vi "create.vi"(8 "error in":errorcluster, 9 "Key":string, 10 "Upload ID":string) -> (0 "error out":errorcluster, 3 "Nominal Client MultiPart Upload":refnum<class "Multipart Upload.lvclass">)   [LabVIEW 2020, in "Multipart Upload.lvclass"]
uses:
  Multipart Upload.lvclass
  Multipart Upload.lvclass/Multipart Upload.ctl
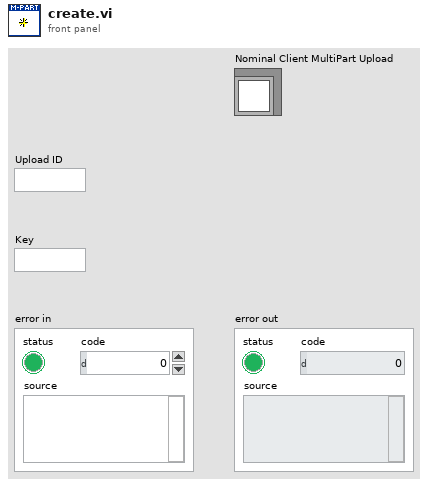
[diagram p1: front panel]
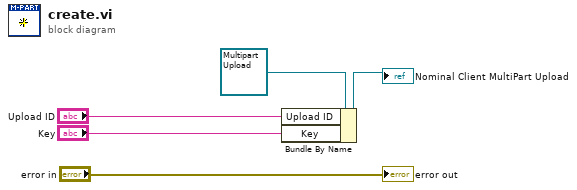
[diagram p0: block diagram]
diagram:
  n1 = Bundle By Name(cluster=refnum<class "Multipart Upload.lvclass"> refnum ("Nominal Client MultiPart Upload"), "Upload ID"="Upload ID", "Key"="Key") -> (→"Nominal Client MultiPart Upload":refnum<class "Multipart Upload.lvclass">)
  "error out" <- "error in"
